vi "Getter Generation tester.vi"() -> ()   [LabVIEW 2020, in "Method Generation.lvlib" / "Getter Generator.lvclass"]
uses:
  Getter Generator.lvclass
panel:
  out "Attributes":map{string, refnum<vi>}(c390)
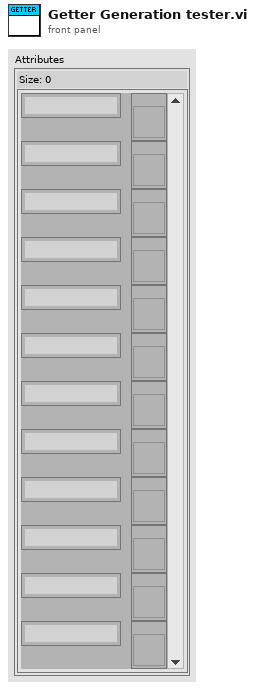
[diagram p1: front panel]
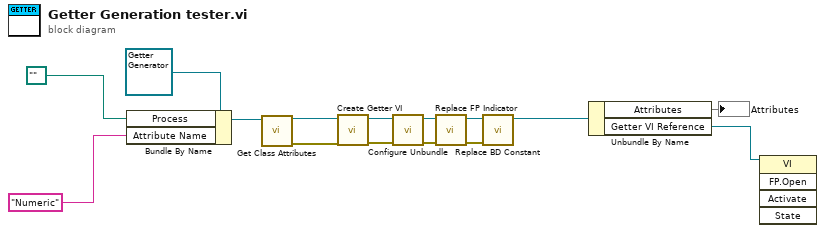
[diagram p0: block diagram]
diagram:
  n1 = Bundle By Name(cluster=refnum<class "Getter Generator.lvclass"> refnum ("New Getter Dialog In"), "Process"=path "", "Attribute Name"="Numeric") -> (w14:refnum<class "Getter Generator.lvclass">)
  n2 = call "Get Class Attributes.vi"("New Getter Dialog In"=w14) -> ("error out"=w10:errorcluster, "New Getter Dialog Out"=w12:refnum<class "Getter Generator.lvclass">)  [unwired: 9 in]
  n3 = call "Create Getter VI.vi"("error in (no error)"=w10, "New Getter Dialog in"=w12) -> ("error out"=w8:errorcluster, "New Getter Dialog out"=w11:refnum<class "Getter Generator.lvclass">)  [unwired: 8 in]
  n4 = call "Configure Unbundle.vi"("error in (no error)"=w8, "Getter Generator in"=w11) -> ("error out"=w3:errorcluster, "Getter Generator out"=w6:refnum<class "Getter Generator.lvclass">)  [unwired: 8 in]
  n5 = call "Replace FP Indicator.vi"("error in (no error)"=w3, "Getter Generator In"=w6) -> ("error out"=w2:errorcluster, "Getter Generator Out"=w5:refnum<class "Getter Generator.lvclass">)  [unwired: 8 in]
  n6 = call "Replace BD Constant.vi"("error in (no error)"=w2, "Getter Generator In"=w5) -> ("Getter Generator Out"=w4:refnum<class "Getter Generator.lvclass">)  [unwired: 8 in, 1 out]
  n7 = Unbundle By Name(w4) -> ("Attributes"=→"Attributes":map{string, refnum<vi>}, "Getter VI Reference"=w7:refnum<vi>)
  n8 = invoke class="VI" method="FP.Open"(reference=w7) -> ()  [unwired: 4 in, 5 out]
